vi "serials db operation.vi"(6 "All serials Data":string[][](array[string]), 7 "SRL DB OP":T2, 8 "error in (no error)":errorcluster, 9 "Status":T1, 10 "Serial":string, 11 "REF":T3) -> (0 "error out":errorcluster, 1 "Serial Status":string, 2 "Fetched Serials":string[][](array[string]), 3 "REF out":T3)   [LabVIEW 2024]
uses:
  CTRLS/REF.ctl
  CTRLS/Main Tabs.ctl
  CTRLS/Open Batch Data.ctl
  CTRLS/DM_Data.ctl
  CTRLS/run statistics.ctl
  CTRLS/System settings.ctl
  CTRLS/Printer Message settings.ctl
  CTRLS/Serials DB Operations Enum.ctl
  CTRLS/Serial status Enum.ctl
  CTRLS/DB operation Selector.ctl
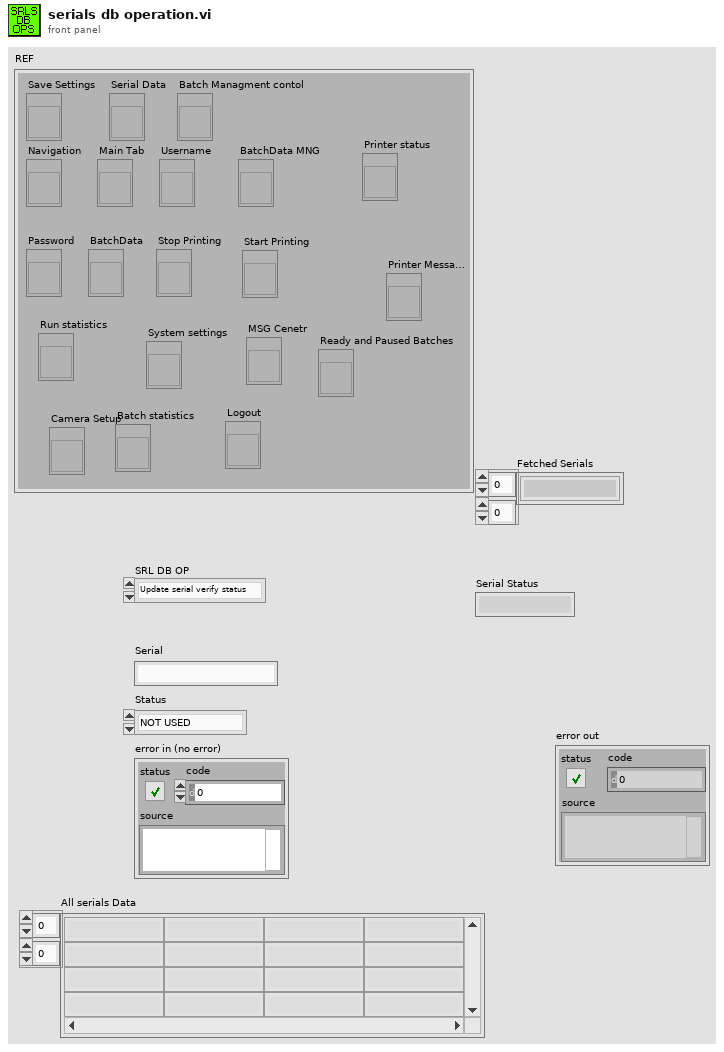
[diagram p1: front panel]
types:
  T1 = typedef "Serial status Enum.ctl" = enum16{"NOT USED", "PRINTED", "ACCEPTED", "REJECTED"}
  T2 = typedef "Serials DB Operations Enum.ctl" = enum16{"Update serial verify status", "Get serials Based on Status", "Insert serials", "Update serial print status", "Get all Batch Serials", "Get Serial Status"}
  T3 = typedef "REF.ctl" = cluster{"Save Settings":refnum<vi>, "Navigation":refnum<vi>, "Main Tab":refnum<vi>, "Password":refnum<vi>, "BatchData":refnum<vi>, "Serial Data":refnum<vi>, "Username":refnum<vi>, "Stop Printing":refnum<vi>, "Run statistics":refnum<vi>, "System settings":refnum<vi>, "Batch Managment contol":refnum<vi>, "Start Printing":refnum<vi>, "BatchData MNG":refnum<vi>, "MSG Cenetr":refnum<vi>, "Printer status":refnum<vi>, "Printer Message Config":refnum<vi>, "Ready and Paused Batches":refnum<vi>, "Camera Setup":refnum<vi>, "Batch statistics":refnum<vi>, "Logout":refnum<vi>}
  T4 = typedef "NI_Database_API.lvlib/Conn ObjectReference.ctl" = refnum<k1>
  T5 = typedef "DB operation Selector.ctl" = enum16{"Select", "Insert", "Update", "Execute select Query", "Execute update query"}
  T6 = cluster{"format string":string, string, "Date and time string":string, "Date and time string":string}
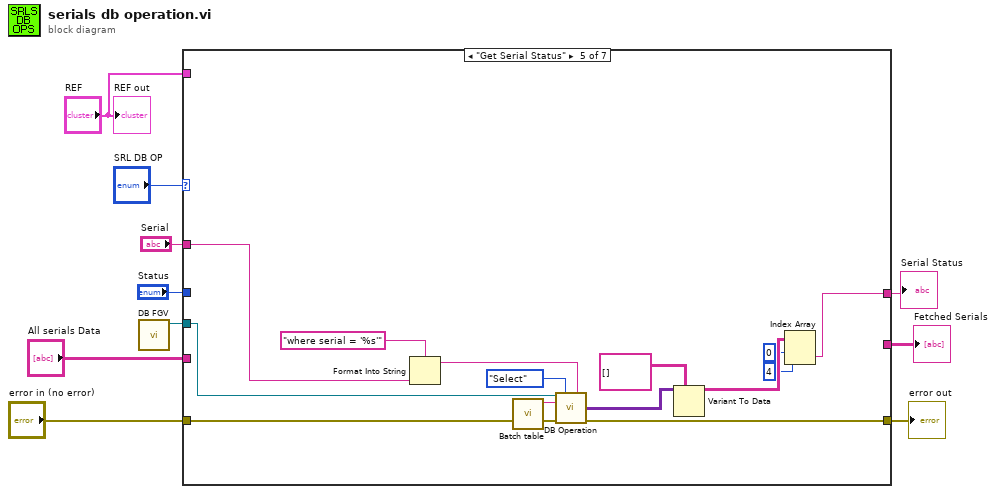
[diagram p0: block diagram]
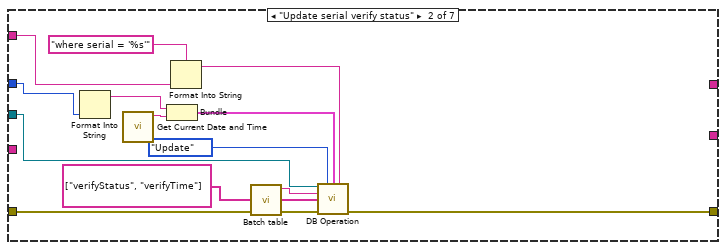
[diagram p3: hidden frame]
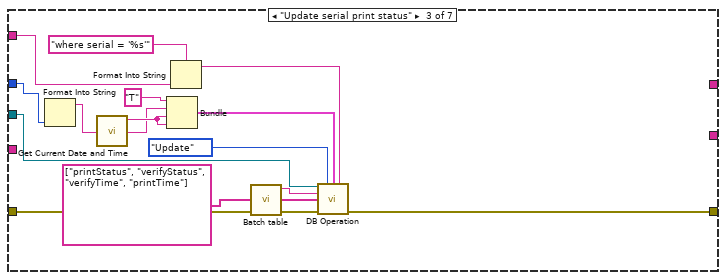
[diagram p4: hidden frame]
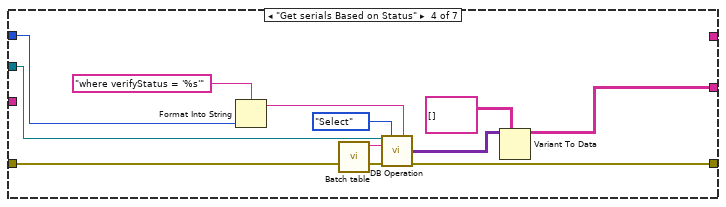
[diagram p5: hidden frame]
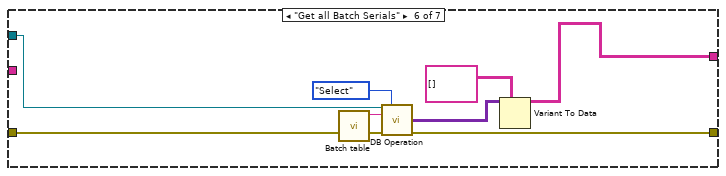
[diagram p6: hidden frame]
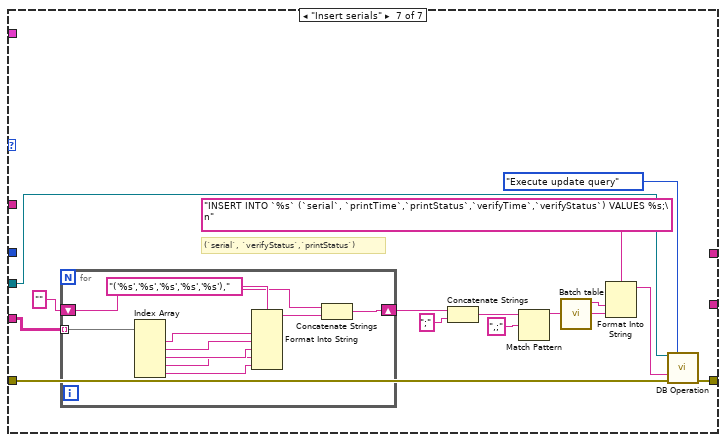
[diagram p7: hidden frame]
diagram:
  n1 = call "DB FGV.vi"() -> ("DB ref"=w9:T4)  [unwired: 11 in]
  n2 = case shown="\"Get Serial Status\"" "SRL DB OP" {
    tunnel: "REF" -> [_ _ _ _ _ _ _]
    tunnel: w9 -> [_ w24 w38 w47 w61 w69 w84]
    tunnel: "Serial" -> [_ w17 w32 _ w54 _ _]
    tunnel: "Status" -> [_ w13 w26 w45 _ _ _]
    tunnel: "error in (no error)" -> [w11 w15 w30 w41 w56 w66 w83]
    tunnel: [w11 w14 w29 w40 w55 w65 w82] -> w4
    tunnel: "All serials Data" -> [_ _ _ _ _ _ w72]
    tunnel: [_ _ _ w39 _ w64 _] -> w2
    tunnel: [_ _ _ _ w50 _ _] -> w1
    frame Default {
    }
    frame "Update serial verify status" {
      n3 = Format Into String(w13) -> (resulting string=w12:string)  [unwired: 3 in, 1 out]
      n4 = call "Get Current Date and Time.vi"() -> ("Date and time string"=w20:string)  [unwired: 11 in]
      n5 = Bundle(w12, "Date and time string"=w20) -> (w19:cluster{string, "Date and time string":string})  [unwired: 1 in]
      n6 = Format Into String(format string="where serial = '%s'", w17) -> (resulting string=w16:string)  [unwired: 2 in, 1 out]
      n7 = call "Batch table.vi"() -> ("Batch table"=w23:string)  [unwired: 11 in]
      n8 = call "DB Operation.vi"("connection reference"=w24, "DB Op Selector"=DB_operation_Selector."Update", "data"=w19, "Condition"=w16, "table"=w23, "columns"=string[] ["verifyStatus", "verifyTime"], "error in (no error)"=w15) -> ("error out"=w14:errorcluster)  [unwired: 6 in, 2 out]
    }
    frame "Update serial print status" {
      n9 = Format Into String(w26) -> (resulting string=w25:string)  [unwired: 3 in, 1 out]
      n10 = call "Get Current Date and Time.vi"() -> ("Date and time string"=w28:string)  [unwired: 11 in]
      n11 = Bundle("format string"="T", w25, "Date and time string"=w28, "Date and time string"=w28) -> (w34:T6)  [unwired: 1 in]
      n12 = Format Into String(format string="where serial = '%s'", w32) -> (resulting string=w31:string)  [unwired: 2 in, 1 out]
      n13 = call "Batch table.vi"() -> ("Batch table"=w37:string)  [unwired: 11 in]
      n14 = call "DB Operation.vi"("connection reference"=w38, "DB Op Selector"=DB_operation_Selector."Update", "data"=w34, "Condition"=w31, "table"=w37, "columns"=string[] ["printStatus", "verifyStatus", "verifyTime", "printTime"], "error in (no error)"=w30) -> ("error out"=w29:errorcluster)  [unwired: 6 in, 2 out]
    }
    frame "Get serials Based on Status" {
      n15 = Format Into String(format string="where verifyStatus = '%s'", w45) -> (resulting string=w44:string)  [unwired: 2 in, 1 out]
      n16 = call "Batch table.vi"() -> ("Batch table"=w49:string)  [unwired: 11 in]
      n17 = call "DB Operation.vi"("connection reference"=w47, "DB Op Selector"=DB_operation_Selector."Select", "Condition"=w44, "table"=w49, "error in (no error)"=w41) -> ("data out"=w42:variant[][], "error out"=w40:errorcluster)  [unwired: 8 in, 1 out]
      n18 = Variant To Data(type=string[][] [], Variant=w42) -> (data=w39:string[][])  [unwired: 1 in, 1 out]
    }
    frame "Get Serial Status" {
      n19 = Format Into String(format string="where serial = '%s'", w54) -> (resulting string=w59:string)  [unwired: 2 in, 1 out]
      n20 = call "Batch table.vi"() -> ("Batch table"=w63:string)  [unwired: 11 in]
      n21 = call "DB Operation.vi"("connection reference"=w61, "DB Op Selector"=DB_operation_Selector."Select", "Condition"=w59, "table"=w63, "error in (no error)"=w56) -> ("data out"=w57:variant[][], "error out"=w55:errorcluster)  [unwired: 8 in, 1 out]
      n22 = Variant To Data(type=string[][] [], Variant=w57) -> (data=w53:string[][])  [unwired: 1 in, 1 out]
      n23 = Index Array(array=w53, index (row)=0, index (col)=4 ("disabled index (col)")) -> (element=w50:string)
    }
    frame "Get all Batch Serials" {
      n24 = call "Batch table.vi"() -> ("Batch table"=w71:string)  [unwired: 11 in]
      n25 = call "DB Operation.vi"("connection reference"=w69, "DB Op Selector"=DB_operation_Selector."Select", "table"=w71, "error in (no error)"=w66) -> ("data out"=w67:variant[][], "error out"=w65:errorcluster)  [unwired: 9 in, 1 out]
      n26 = Variant To Data(type=string[][] [], Variant=w67) -> (data=w64:string[][])  [unwired: 1 in, 1 out]
    }
    frame "Insert serials" {
      # "(`serial`, `verifyStatus`,`printStatus`)"
      n27 = for {
        shift-right: [w92] -> w78
        shift-left: "" -> [w94]
        tunnel: w72 -> [w91] mode=indexing
        n28 = Index Array(array=w91) -> (element #1=w90:string, element #2=w89:string, element #3=w88:string, element #4=w87:string, element #5=w86:string)  [unwired: 5 in]
        n29 = Format Into String(format string="('%s','%s','%s','%s','%s'),", w90, w89, w88, w87, w86) -> (resulting string=w93:string)  [unwired: 2 in, 1 out]
        n30 = Concatenate Strings(w94, w93) -> (w92:string)
      }
      n31 = Concatenate Strings(w78, ";" ("string")) -> (w76:string)
      n32 = Match Pattern(string=w76, regular expression=",;") -> (before substring=w74:string)  [unwired: 1 in, 3 out]
      n33 = call "Batch table.vi"() -> ("Batch table"=w73:string)  [unwired: 11 in]
      n34 = Format Into String(format string="INSERT INTO `%s` (`serial`, `printTime`,`printStatus`,`verifyTime`,`verifyStatus`) VALUES %s;\n", w73, w74) -> (resulting string=w79:string)  [unwired: 2 in, 1 out]
      n35 = call "DB Operation.vi"("connection reference"=w84, "DB Op Selector"=DB_operation_Selector."Execute update query", "SQL Query"=w79, "error in (no error)"=w83) -> ("error out"=w82:errorcluster)  [unwired: 9 in, 2 out]
    }
  }
  "error out" <- w4
  "Fetched Serials" <- w2
  "Serial Status" <- w1
  "REF out" <- "REF"
